vi "Add Client.vi"(8 "error in (no error)":errorcluster, 10 "Client":refnum<class "TCP Client.lvclass">, 11 "TCP Server in":refnum<class "TCP Server.lvclass">) -> (0 "error out":errorcluster, 3 "TCP Server out":refnum<class "TCP Server.lvclass">)   [LabVIEW 2020, in "Stream-TCP.lvlib" / "TCP Server.lvclass"]
uses:
  TCP Server.lvclass
  TCP Client/TCP Client.lvclass
  TCP Server.lvclass/TCP Server.ctl
  Server Connection Callback.vi
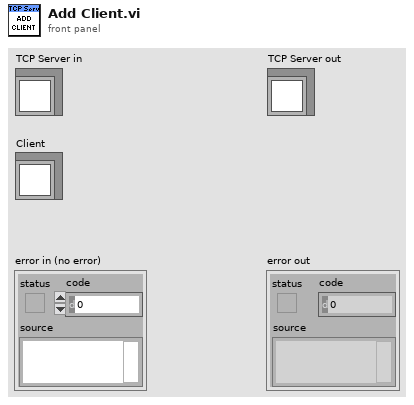
[diagram p1: front panel]
types:
  T1 = typedef "Stream-TCP.lvlib/TCP Server.lvclass/Ref Data.ctl" = cluster{"Listener":refnum<k5>, "Clients":refnum<class "TCP Client.lvclass">[], "Server Loop":bool}
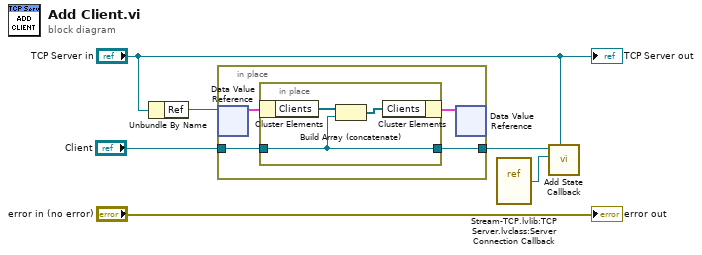
[diagram p0: block diagram]
diagram:
  n1 = Unbundle By Name("TCP Server in") -> ("Ref"=w5:refnum<data-value>)
  n2 = in-place {
    in-place-border: "Client" -> [w8]
    in-place-border: [w7] -> w3
    n3 = in-place-dvr #1(w5) -> (w10:T1)  [unwired: 1 out]
    n4 = in-place {
      in-place-border: w8 -> [w11]
      in-place-border: [w11] -> w7
      n5 = in-place-cluster #2(w10) -> ("Clients"=w13:refnum<class "TCP Client.lvclass">[])
      n6 = Build Array (concatenate)(w13, w11) -> (w12:refnum<class "TCP Client.lvclass">[])
      n7 = in-place-cluster #2("Clients"=w12) -> (w9:T1)
    }
    n8 = in-place-dvr #1(w9) -> ()  [unwired: 2 out]
  }
  n9 = vi-ref "Stream-TCP.lvlib:TCP Server.lvclass:Server Connection Callback.vi"() -> (w1:refnum<vi>)
  n10 = call-dynamic "Add State Callback.vi"("Owner (None)"="TCP Server in", "Callback"=w1, "Connection in"=w3) -> ()  [unwired: 7 in, 2 out]
  "error out" <- "error in (no error)"
  "TCP Server out" <- "TCP Server in"
